vi "Parse Project for items.vi"(8 "error in":errorcluster, 11 "Project":refnum<vi>) -> (0 "error out":errorcluster, 3 "Items":T1[](array[typedef]))   [LabVIEW 2020, in "ConstantErrorsMaker.lvlib"]
uses:
  ConstantErrorsMaker.lvlib
  Selection Info--cluster.ctl
  Selection Type--enum.ctl
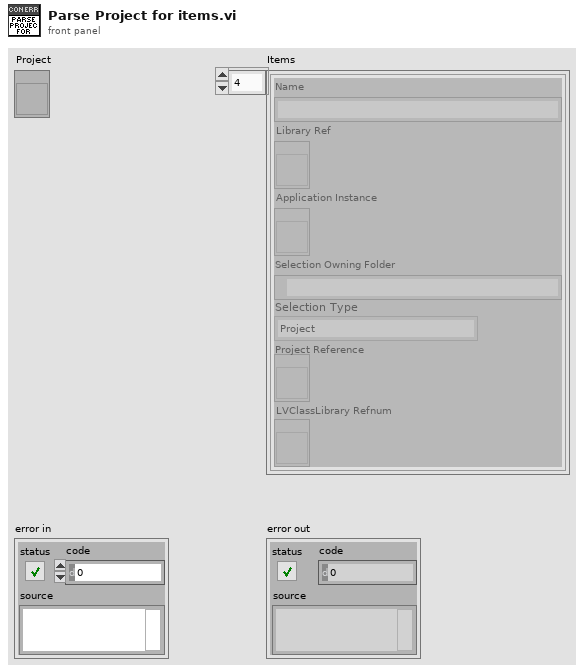
[diagram p1: front panel]
types:
  T1 = typedef "ConstantErrorsMaker.lvlib/Selection Info--cluster.ctl" = cluster{"Name":string, "Library Ref":refnum<vi>, "Application Instance":refnum<vi>, "Selection Owning Folder":path, "Selection Type":T2, "Project Reference":refnum<vi>, "LVClassLibrary Refnum":refnum<vi>}
  T2 = typedef "ConstantErrorsMaker.lvlib/Selection Type--enum.ctl" = enum16{"Project", "Library", "Class"}
  T3 = enum32{"invalid lock state", "Not Locked", "Locked (No Password)", "Password-protected"}
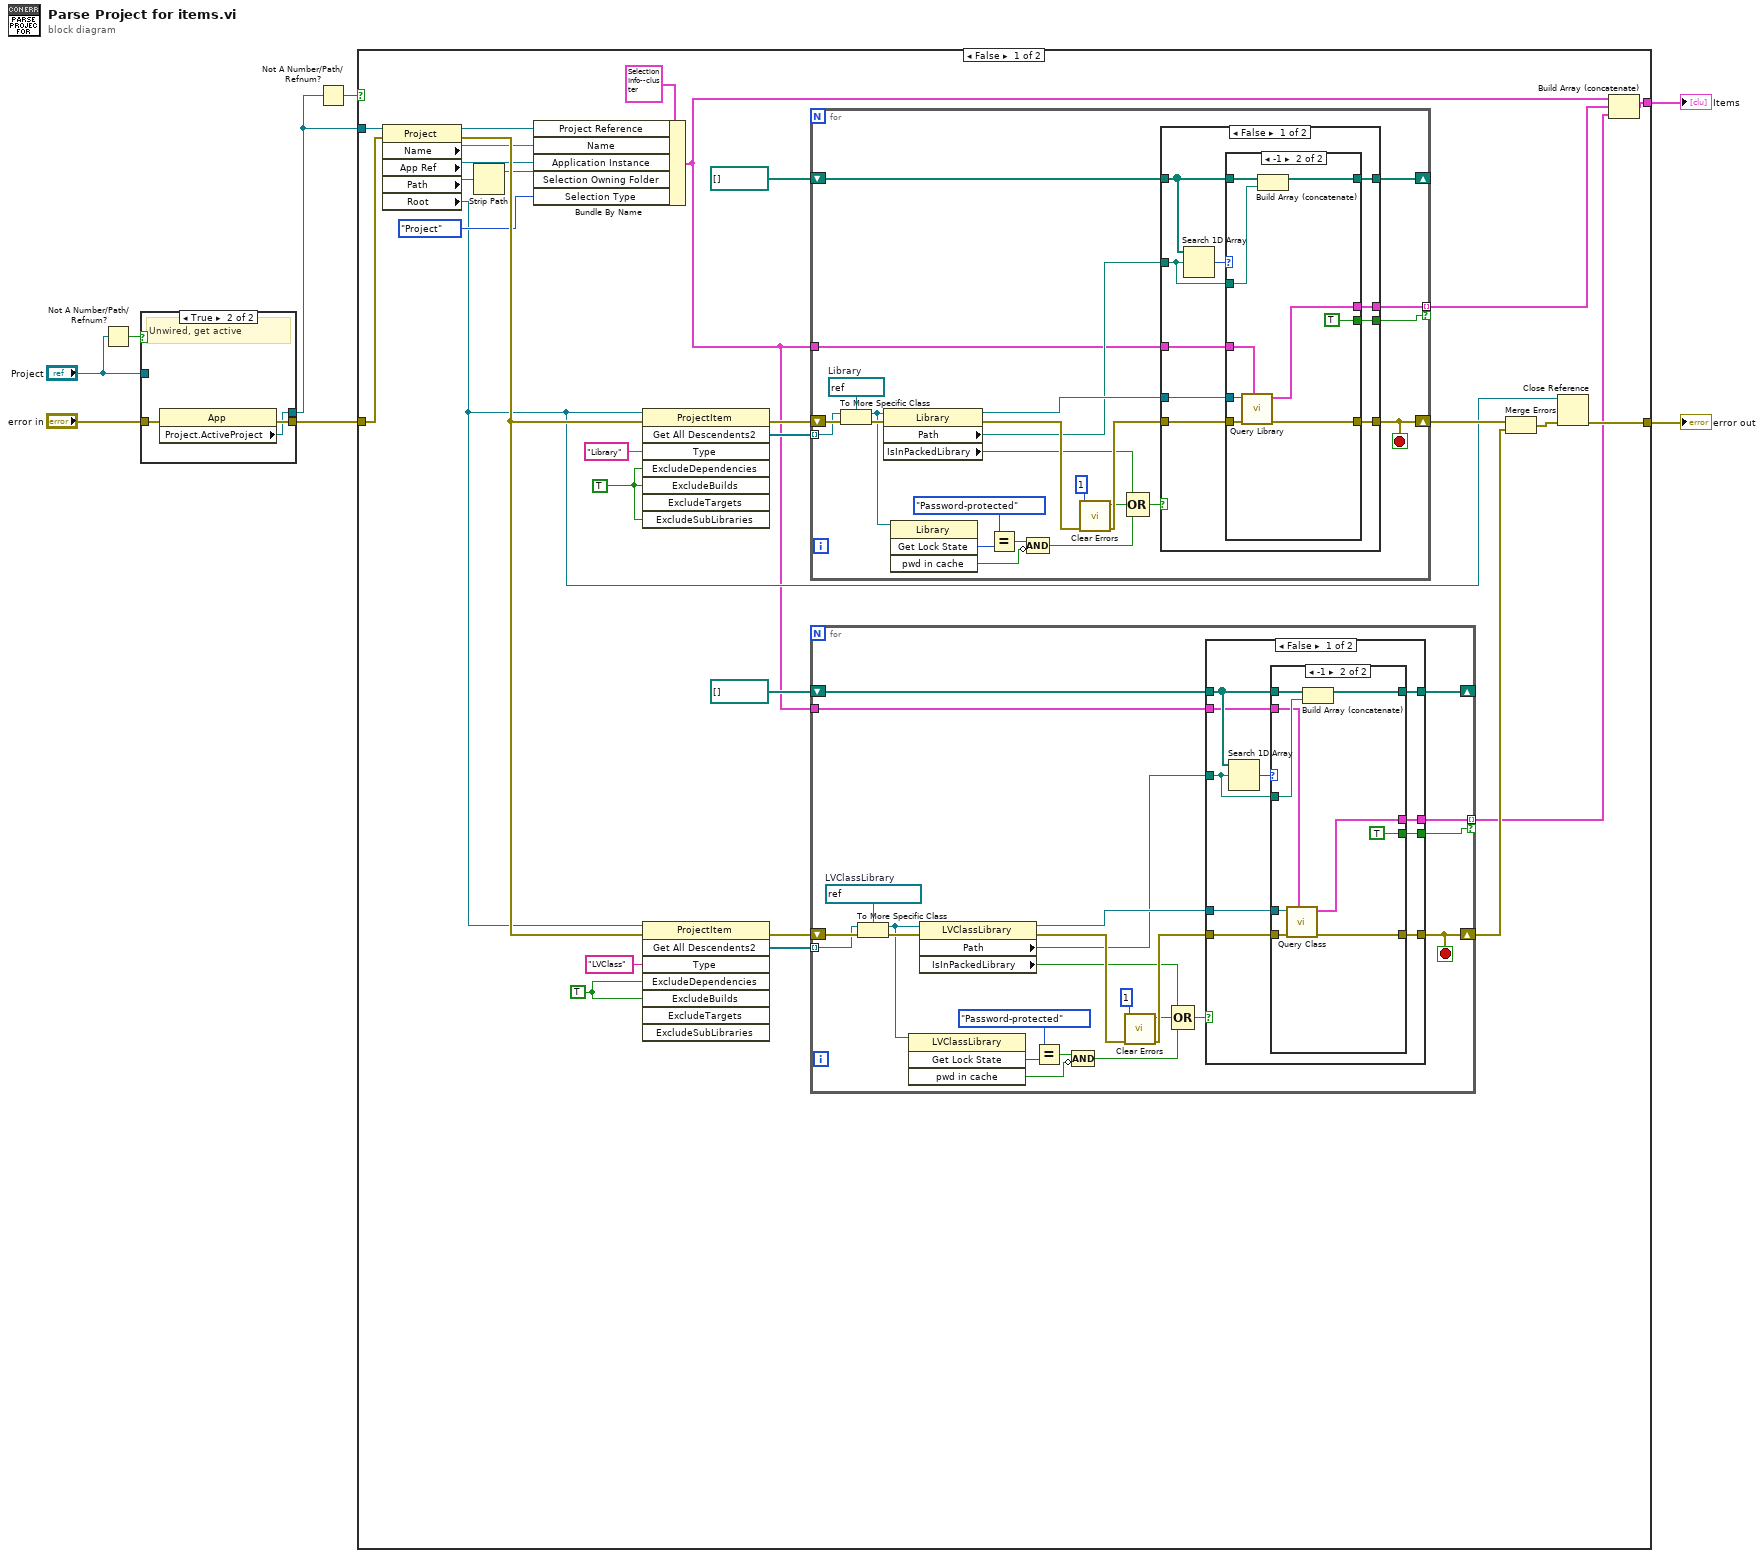
[diagram p0: block diagram]
diagram:
  n1 = Not A Number/Path/Refnum?(number/path/refnum="Project") -> (NaN/Path/Refnum?=w3:bool)
  n2 = case shown="True" w3 {
    tunnel: "Project" -> [w9 _]
    tunnel: "error in" -> [w10 w13]
    tunnel: [w9 w11] -> w2
    tunnel: [w10 w12] -> w6
    frame False {
    }
    frame True {
      # "Unwired, get active"
      n3 = property class="App"(error in=w13) -> (error out=w12:errorcluster, "Project.ActiveProject"=w11:refnum<vi>)  [unwired: 1 in, 1 out]
    }
  }
  n4 = Not A Number/Path/Refnum?(number/path/refnum=w2) -> (NaN/Path/Refnum?=w1:bool)
  n5 = case shown="False" w1 {
    tunnel: w6 -> [w40 w137]
    tunnel: [w39 w137] -> w7
    tunnel: w2 -> [w23 _]
    tunnel: [w21 _] -> w4
    frame False {
      w16 = TRUE
      w27 = TRUE
      n6 = property class="Project"(reference=w23, error in=w40) -> (reference out=w26:refnum<vi>, error out=w37:errorcluster, "Name"=w30:string, "App Ref"=w24:refnum<vi>, "Path"=w28:path, "Root"=w18:refnum<vi>)
      n7 = Strip Path(path=w28) -> (stripped path=w25:path)  [unwired: 1 out]
      n8 = Bundle By Name(cluster=T1 {"Name"="", "Library Ref"=refnum, "Application Instance"=refnum, "Selection Owning Folder"=path "", "Selection Type"=enum."Project", "Project Reference"=refnum, "LVClassLibrary Refnum"=refnum} ("Selection Info"), "Project Reference"=w26, "Name"=w30, "Application Instance"=w24, "Selection Owning Folder"=w25, "Selection Type"=Selection_Type--enum."Project") -> (w14:T1)
      n9 = invoke class="ProjectItem" method="Get All Descendents2"(reference=w18, error in=w37, "Type"="Library", "ExcludeDependencies"=w27, "ExcludeBuilds"=w27, "ExcludeSubLibraries"=w27) -> (error out=w42:errorcluster, "Get All Descendents2"=w33:refnum<vi>[])  [unwired: 2 in, 6 out]
      n10 = invoke class="ProjectItem" method="Get All Descendents2"(reference=w18, error in=w37, "Type"="LVClass", "ExcludeDependencies"=w16, "ExcludeBuilds"=w16) -> (error out=w38:errorcluster, "Get All Descendents2"=w20:refnum<vi>[])  [unwired: 3 in, 6 out]
      n11 = for {
        tunnel: w33 -> [w108] mode=indexing
        shift-right: [w111] -> w41
        shift-left: w42 -> [w113]
        tunnel: [w106] -> w22 mode=indexing if=w95
        shift-right: [w103] -> _
        shift-left: path[] [] -> [w104]
        tunnel: w14 -> [w90]
        stop <- w111 stop-if-true
        w107 = refnum<vi> refnum  # Library
        n12 = To More Specific Class(target class=w107, reference=w108, error in=w113) -> (specific class reference=w101:refnum<vi>, error out=w112:errorcluster)
        n13 = property class="Library"(reference=w101, error in=w112) -> (reference out=w105:refnum<vi>, error out=w110:errorcluster, "Path"=w94:path, "IsInPackedLibrary"=w102:bool)
        n14 = invoke class="Library" method="Get Lock State"(reference=w101) -> ("Get Lock State"=w100:T3, "pwd in cache"=w97:bool)  [unwired: 3 in, 2 out]
        n15 = Equal?(x=T3."Password-protected", y=w100) -> (x = y?=w98:bool)
        n16 = Compound Arithmetic op=AND(w98, invert w97) -> (w96:bool)
        n17 = call <vilib>:"Clear Errors.vi"("error in (no error)"=w110, "specific error code to clear (0: all)"=1) -> ("error out"=w109:errorcluster, "specific error cleared?"=w92:bool)  [unwired: 4 in]
        n18 = Compound Arithmetic op=OR(w102, w92, w96) -> (w91:bool)
        n19 = case shown="False" w91 {
          tunnel: [w123 w136] -> w111
          tunnel: [w121 _] -> w106
          tunnel: w105 -> [w120 _]
          tunnel: w104 -> [w118 w135]
          tunnel: [w117 w135] -> w103
          tunnel: w94 -> [w116 _]
          tunnel: w109 -> [w122 w136]
          tunnel: [w115 _] -> w95
          tunnel: w90 -> [w114 _]
          frame False {
            n20 = Search 1D Array(1D array=w118, element=w116) -> (index of element=w119:i32)  [unwired: 1 in]
            n21 = case shown="-1" w119 {
              tunnel: [w125 w134] -> w123
              tunnel: [_ w132] -> w121
              tunnel: w122 -> [w125 w133]
              tunnel: w120 -> [_ w131]
              tunnel: w118 -> [w124 w130]
              tunnel: [w124 w128] -> w117
              tunnel: w116 -> [_ w129]
              tunnel: [_ TRUE] -> w115
              tunnel: w114 -> [_ w126]
              frame Default {
              }
              frame -1 {
                n22 = call "Query Library.vi"("Selection Info"=w126, "error in"=w133, "Library"=w131) -> ("error out"=w134:errorcluster, "Library Info"=w132:T1)  [unwired: 6 in, 1 out]
                n23 = Build Array (concatenate)(w130, w129) -> (w128:path[])
              }
            }
          }
          frame True {
            # "If Item is inside a PPL or it is password protected we can't create any error or constants\nAdditionally, if the error -1 pops out, it means it is an unsaved or non present library"
          }
        }
      }
      n24 = for {
        tunnel: w20 -> [w61] mode=indexing
        shift-right: [w64] -> w35
        shift-left: w38 -> [w66]
        tunnel: [w59] -> w15 mode=indexing if=w48
        shift-right: [w56] -> _
        shift-left: path[] [] -> [w57]
        tunnel: w14 -> [w43]
        stop <- w64 stop-if-true
        w60 = refnum<vi> refnum  # LVClassLibrary
        n25 = To More Specific Class(target class=w60, reference=w61, error in=w66) -> (specific class reference=w54:refnum<vi>, error out=w65:errorcluster)
        n26 = invoke class="LVClassLibrary" method="Get Lock State"(reference=w54) -> ("Get Lock State"=w53:T3, "pwd in cache"=w50:bool)  [unwired: 3 in, 2 out]
        n27 = property class="LVClassLibrary"(reference=w54, error in=w65) -> (reference out=w58:refnum<vi>, error out=w63:errorcluster, "Path"=w47:path, "IsInPackedLibrary"=w55:bool)
        n28 = Equal?(x=T3."Password-protected", y=w53) -> (x = y?=w51:bool)
        n29 = Compound Arithmetic op=AND(w51, invert w50) -> (w49:bool)
        n30 = call <vilib>:"Clear Errors.vi"("error in (no error)"=w63, "specific error code to clear (0: all)"=1) -> ("error out"=w62:errorcluster, "specific error cleared?"=w45:bool)  [unwired: 4 in]
        n31 = Compound Arithmetic op=OR(w55, w45, w49) -> (w44:bool)
        n32 = case shown="False" w44 {
          tunnel: [w76 w89] -> w64
          tunnel: [w74 _] -> w59
          tunnel: w58 -> [w73 _]
          tunnel: w57 -> [w71 w88]
          tunnel: [w70 w88] -> w56
          tunnel: w47 -> [w69 _]
          tunnel: w62 -> [w75 w89]
          tunnel: [w68 _] -> w48
          tunnel: w43 -> [w67 _]
          frame False {
            n33 = Search 1D Array(1D array=w71, element=w69) -> (index of element=w72:i32)  [unwired: 1 in]
            n34 = case shown="-1" w72 {
              tunnel: [w78 w87] -> w76
              tunnel: [_ w85] -> w74
              tunnel: w75 -> [w78 w86]
              tunnel: w73 -> [_ w84]
              tunnel: w71 -> [w77 w83]
              tunnel: [w77 w81] -> w70
              tunnel: w69 -> [_ w82]
              tunnel: [_ TRUE] -> w68
              tunnel: w67 -> [_ w79]
              frame Default {
              }
              frame -1 {
                n35 = call "Query Class.vi"("Selection Info"=w79, "error in"=w86, "LVClassLibrary Refnum"=w84) -> ("error out"=w87:errorcluster, "Class Info"=w85:T1)  [unwired: 6 in, 1 out]
                n36 = Build Array (concatenate)(w83, w82) -> (w81:path[])
              }
            }
          }
          frame True {
            # "If Item is inside a PPL or it is password protected we can't create any error or constants\nAdditionally, if the error -1 pops out, it means it is an unsaved or non present library"
          }
        }
      }
      n37 = Merge Errors(w41, w35) -> (w36:errorcluster)
      n38 = Close Reference(reference=w18, error in (no error)=w36) -> (error out=w39:errorcluster)
      n39 = Build Array (concatenate)(w14, w22, w15) -> (w21:T1[])
    }
    frame True {
    }
  }
  "error out" <- w7
  "Items" <- w4
